vi "Incomplete Beta Function.vi"(9 "a":dbl=1.0 format="%.2f", 10 "y":dbl format="%.2f", 11 "x":dbl format="%.2f") -> (3 "b(x, y, a)":dbl format="%.2f")   [LabVIEW 2020, in "NI_Gmath.lvlib"]
doc: "Evaluates the beta function and regularized incomplete beta function. You must manually select the polymorphic instance you want to use."
uses:
  NI_Gmath.lvlib
  <resource>/lvanlys.dll
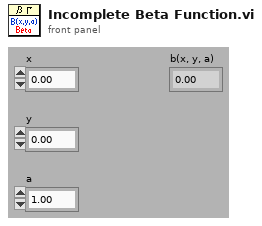
[diagram p1: front panel]
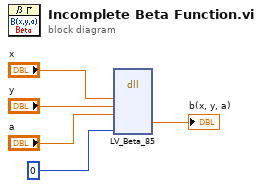
[diagram p0: block diagram]
diagram:
  n1 = dll-call lib="C:/Program Files (x86)/National Instruments/LabVIEW 2020/resource/lvanlys.*" fn="LV_Beta_85"("x"="x", "y"="y", "a"="a", "funcType"=0) -> ("beta(x,y,a)"=→"b(x, y, a)":dbl)  [unwired: 9 in, 2 out]
